vi "MotorBlock_PI.vi"(0 "P":dbl, 3 "STOP":bool, 5 "Value":dbl, 7 "Custom FPGA Reference Out":refnum<k20>, 9 "Speed\n (Lower than 900 counts/s)":dbl, 11 "error in (no error)":errorcluster, 12 "Enum":T2(ring), 13 "Motor":T1(ring), 14 "(Antihorario) Sentido (Horario)":bool) -> (4 "Waveform \nChart":dbl[][](graph), 10 "Custom FPGA Reference Out 2":refnum<k20>, 15 "error out":errorcluster)   [LabVIEW 2017]
uses:
  <vilib>/myRIO/Common/Instrument Driver Framework/myRIO v1.0/Encoder/typedefs/Encoder Signal Mode.ctl
  <vilib>/Platform/TimedLoop/XDataNode/timing_clust.ctl
  <vilib>/Platform/TimedLoop/XDataNode/nitl_modes.ctl
  <vilib>/Platform/TimedLoop/XDataNode/wakeup.ctl
  <vilib>/myRIO/Common/Instrument Driver Framework/myRIO v1.0/UART/vis/myRIO v1.0 Close UART.vi
  <vilib>/Utility/error.llb/Error Cluster From Error Code.vi
  <vilib>/myRIO/Common/Instrument Driver Framework/myRIO v1.0/Encoder/vis/myRIO v1.0 Read Encoder.vi
  <vilib>/myRIO/Common/Instrument Driver Framework/myRIO v1.0/DIO/vis/myRIO v1.0 Write DIO.vi
  <vilib>/myRIO/Common/Instrument Driver Framework/myRIO v1.0/PWM/vis/myRIO v1.0 Write PWM.vi
  <vilib>/myRIO/Common/Instrument Driver Framework/Utilities/vis/FPGA Ref Manager.vi
  <vilib>/myRIO/Common/Instrument Driver Framework/myRIO v1.0/myRIO v1.0 Reset FPGA.vi
  <vilib>/myRIO/Common/Instrument Driver Framework/myRIO v1.0/IRQ/vis/myRIO v1.0 IRQ Info FGV.vi
  <vilib>/myRIO/Common/Instrument Driver Framework/myRIO v1.0/IRQ/vis/myRIO v1.0 Timer IRQ Info FGV.vi
  <vilib>/myRIO/Common/Instrument Driver Framework/myRIO v1.0/IRQ/vis/myRIO v1.0 ISR Agent.vi
  <vilib>/Platform/TimedLoop/XDataNode/XDataNode.xnode
  <vilib>/myRIO/Instrument Drivers/Utilities/Utilities.lvlib
  <vilib>/myRIO/Instrument Drivers/Onboard IO/PWM/PWM.lvlib
  <vilib>/myRIO/Instrument Drivers/Onboard IO/DIO/DIO.lvlib
  <vilib>/myRIO/Instrument Drivers/Onboard IO/Encoder/Encoder.lvlib
  <vilib>/Platform/TimedLoop/XDataNode/XDNodeRunTimeDep.lvlib
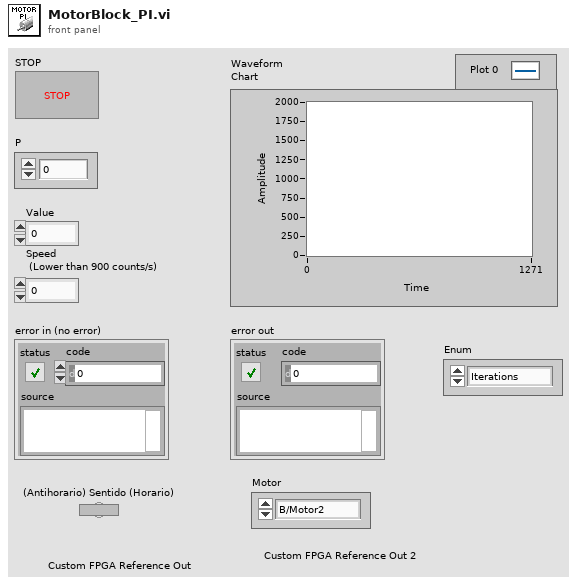
[diagram p1: front panel]
types:
  T1 = enum16{"B/Motor2", "B/Motor1", "A/Motor2", "A/Motor1"}
  T2 = enum16{"Iterations", "Rotations", "Counts", "Degrees", "Time"}
  T3 = typedef "Encoder Signal Mode.ctl" = enum16{"Quadrature phase signal", "Step and direction signal"}
  T4 = typedef "XDNodeRunTimeDep.lvlib/timing_clust.ctl" = cluster{"Expected End [f-1]":u64, "Actual End [f-1]":u64, "Finished Late? [f-1]":bool, "Expected End [i-1]":u64, "Actual End [i-1]":u64, "Finished Late? [i-1]":bool, "Expected Start [i]":u64, "Actual Start [i]":u64, "Expected Start [f]":u64, "Actual Start [f]":u64, "Source Name":string, "Structure Name":string, "Period":i64, "Deadline":i64, "Offset":i64, "Start":i64, "Priority":i32, "Timeout":i32, "Mode":T5, "Wakeup Reason":T6, "Error":errorcluster, "Source Type":string, "Secondary Source Type":string, "Global End Time":u64, "Global Start Time":u64, "Frame Duration":u64, "Iteration Duration":u64, "Assigned CPU":i32, "I/O Scan Engine Mode":u32}
  T5 = typedef "XDNodeRunTimeDep.lvlib/nitl_modes.ctl" = enum32{"No Change", "Process missed periods, maintain original phase", "Discard missed periods, maintain original phase", "Process missed periods, ignore original phase", "Discard missed periods, ignore original phase"}
  T6 = typedef "XDNodeRunTimeDep.lvlib/wakeup.ctl" = enum32{"Normal", "Aborted", "Asynchronous wakeup", "Timing source error", "Timed loop error", "Timeout"}
  T7 = typedef "Encoder.lvlib/Encoder Reference.ctl" = cluster{"myRIO Reference":T8, "Encoder Channels Enum":T12}
  T8 = typedef "myRIO Generic Hardware Reference.ctl" = cluster{"myRIO Model":T9, "myRIO Hardware Reference":T10}
  T9 = typedef "Hardware Version Enum.ctl" = enum16{"Unknown", "myRIO-1900", "myRIO-1950", "roboRIO", "NI ELVIS RIO CM"}
  T10 = typedef "myRIO v1.0 Reference.ctl" = cluster{"Generic FPGA Reference":T11, "Allow multiple opens":bool}
  T11 = typedef "Generic FPGA Reference.ctl" = refnum<k20>
  T12 = typedef "Encoder Channels Enum.ctl" = enum16{"Not Connected", "C/ENC0", "C/ENC1", "A/ENC", "B/ENC", "DIO/ENC0", "DIO/ENC1", "DIO/ENC2", "DIO/ENC3", "DIO/ENC4"}
  T13 = typedef "DIO.lvlib/DIO Reference.ctl" = cluster{"myRIO Reference":T8, "DIO Channels List":T14}
  T14 = typedef "DIO Channels List.ctl" = T15[]
  T15 = typedef "DIO Channels Enum.ctl" = enum16{"Not Connected", "C/DIO0", "C/DIO1", "C/DIO2", "C/DIO3", "C/DIO4", "C/DIO5", "C/DIO6", "C/DIO7", "A/DIO0", "A/DIO1", "A/DIO2", "A/DIO3", "A/DIO4", "A/DIO5", "A/DIO6", "A/DIO7", "A/DIO8", "A/DIO9", "A/DIO10", "A/DIO11", "A/DIO12", "A/DIO13", "A/DIO14", "A/DIO15", "B/DIO0", "B/DIO1", "B/DIO2", "B/DIO3", "B/DIO4", "B/DIO5", "B/DIO6", "B/DIO7", "B/DIO8", "B/DIO9", "B/DIO10", "B/DIO11", "B/DIO12", "B/DIO13", "B/DIO14", "B/DIO15", "LED0", "LED1", "LED2", "LED3", "Button0", "DIO/DIO0", "DIO/DIO1", "DIO/DIO2", "DIO/DIO3", "DIO/DIO4", "DIO/DIO5", "DIO/DIO6", "DIO/DIO7", "DIO/DIO8", "DIO/DIO9", "SPI/CS0", "SPI/CS1", "SPI/CS2", "SPI/CS3", "LED RADIO (Green)", "LED RADIO (Red)", "LED COMM (Green)", "LED COMM (Red)", "LED MODE (Green)", "LED MODE (Red)"}
  T16 = typedef "PWM.lvlib/PWM Reference.ctl" = cluster{"myRIO Reference":T8, "PWM Channels Enum":T17, "PWM Configuration":T18}
  T17 = typedef "PWM Channels Enum.ctl" = enum16{"Not Connected", "C/PWM0", "C/PWM1", "A/PWM0", "A/PWM1", "A/PWM2", "B/PWM0", "B/PWM1", "B/PWM2", "PWM/PWM0", "PWM/PWM1", "PWM/PWM2", "PWM/PWM3", "PWM/PWM4", "PWM/PWM5", "PWM/PWM6", "PWM/PWM7", "PWM/PWM8", "PWM/PWM9"}
  T18 = typedef "PWM.lvlib/PWM Configuration.ctl" = cluster{"Frequency":dbl, "Duty Cycle":dbl}
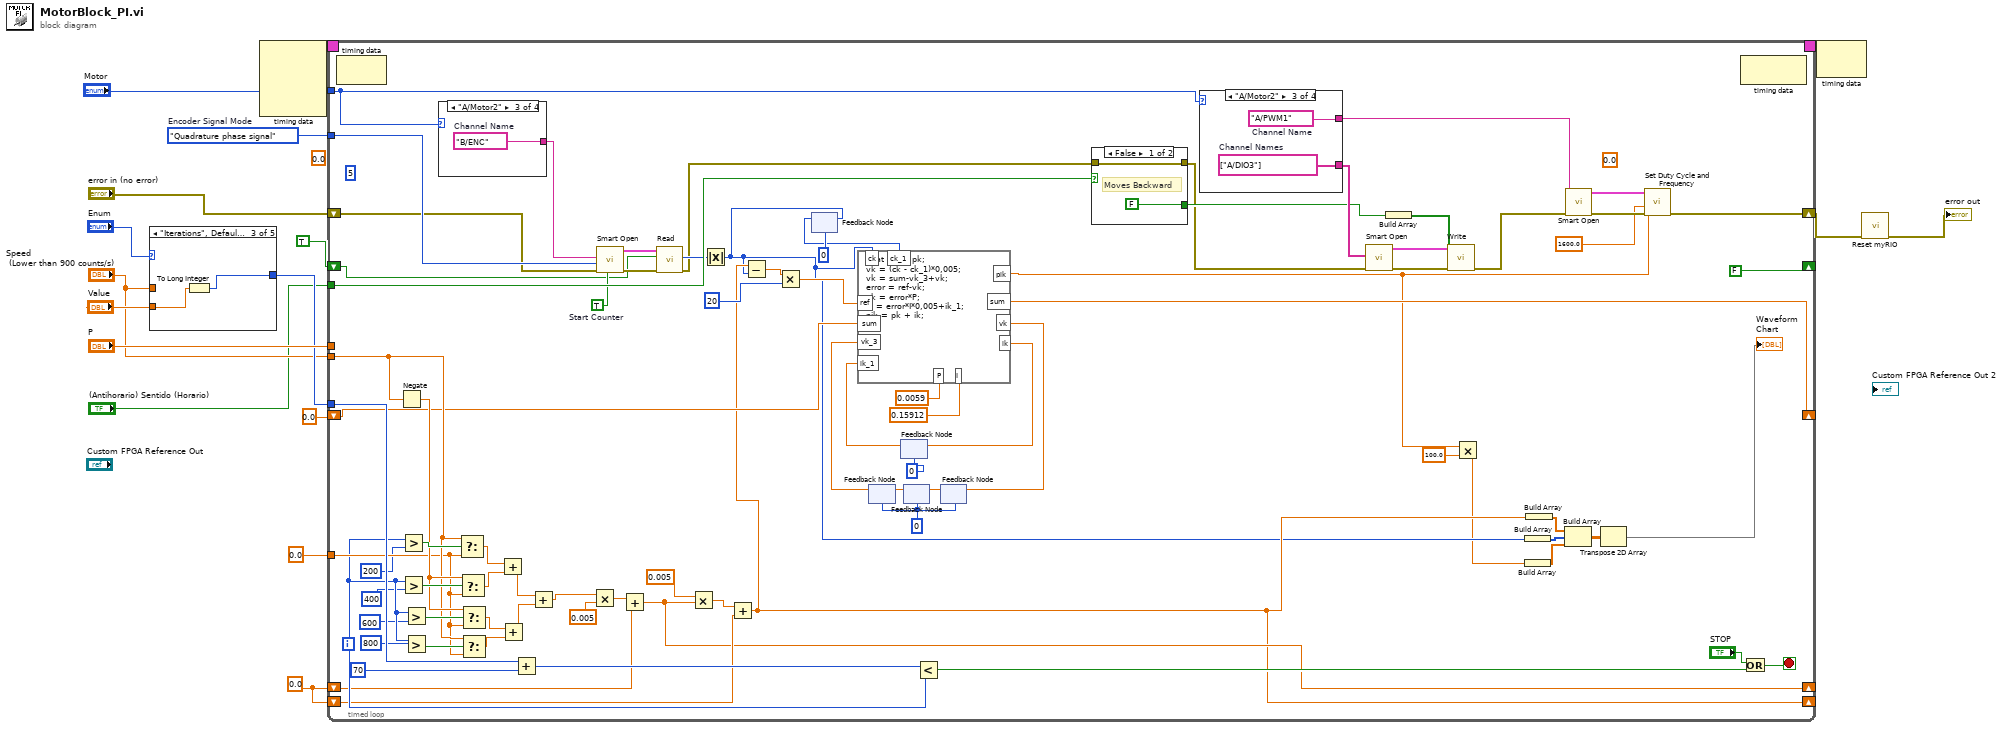
[diagram p0: block diagram]
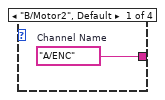
[diagram p2: hidden frame]
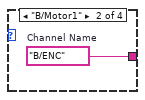
[diagram p3: hidden frame]
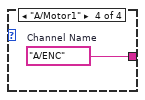
[diagram p4: hidden frame]
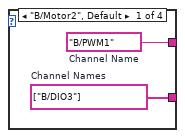
[diagram p5: hidden frame]
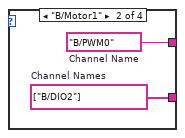
[diagram p6: hidden frame]
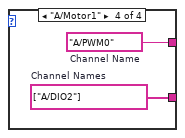
[diagram p7: hidden frame]
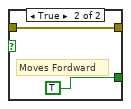
[diagram p8: hidden frame]
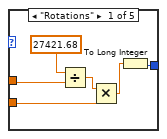
[diagram p9: hidden frame]
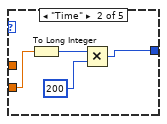
[diagram p10: hidden frame]
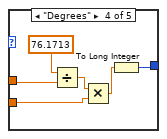
[diagram p11: hidden frame]
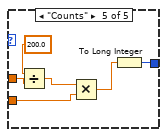
[diagram p12: hidden frame]
diagram:
  w1 = 0.0
  w5 = Encoder_Signal_Mode."Quadrature phase signal"  # Encoder Signal Mode
  (unwired) 0.0
  n1 = case shown="\"Iterations\", Default" "Enum" {
    tunnel: "Value" -> [w19 w24 w29 w30 w37]
    tunnel: "Speed\n (Lower than 900 counts/s)" -> [w20 _ _ w33 w40]
    tunnel: [w18 w26 w28 w35 w41] -> w11
    frame "Rotations" {
      n2 = Divide(x=27421.68 ("y"), y=w20) -> (x/y=w23:dbl)
      n3 = Multiply(x=w23, y=w19) -> (x*y=w21:dbl)
      n4 = To Long Integer(number=w21) -> (32bit integer=w18:i32)
    }
    frame "Time" {
      n5 = To Long Integer(number=w24) -> (32bit integer=w25:i32)
      n6 = Multiply(x=w25, y=200) -> (x*y=w26:i32)
    }
    frame "Iterations", Default {
      n7 = To Long Integer(number=w29) -> (32bit integer=w28:i32)
    }
    frame "Degrees" {
      n8 = Divide(x=76.1713 ("y"), y=w33) -> (x/y=w31:dbl)
      n9 = Multiply(x=w31, y=w30) -> (x*y=w34:dbl)
      n10 = To Long Integer(number=w34) -> (32bit integer=w35:i32)
    }
    frame "Counts" {
      n11 = Divide(x=200.0, y=w40) -> (x/y=w38:dbl)
      n12 = Multiply(x=w38, y=w37) -> (x*y=w36:dbl)
      n13 = To Long Integer(number=w36) -> (32bit integer=w41:i32)
    }
  }
  n14 = node-c288() -> (w4:T4)  [unwired: 4 in]
  n15 = timed-loop {
    shift-right: [w66] -> _
    shift-left: 0.0 -> [w65]
    shift-right: [FALSE] -> _
    shift-left: TRUE -> [w99]
    tunnel: "P" -> [_]
    tunnel: "Speed\n (Lower than 900 counts/s)" -> [w91]
    shift-right: [w112] -> w6
    shift-left: "error in (no error)" -> [w96]
    tunnel: w11 -> [w119]
    tunnel: "(Antihorario) Sentido (Horario)" -> [w123]
    tunnel: "Motor" -> [w101]
    tunnel: w5 -> [w97]
    timing: w4 -> [_]
    timing-out: [_] -> w3
    tunnel: 0.0 ("f") -> [w89]
    shift-right: [w52] -> _
    shift-left: w1 -> [w54]
    shift-right: [w47] -> _
    shift-left: w1 -> [w53]
    i -> [w77]
    stop <- w120 stop-if-true
    (unwired) 0.0 ("Duty Cycle")
    w72 = 0
    w104 = TRUE  # Start Counter
    (unwired) 5
    n16 = node-c288() -> ()  [unwired: 1 in, 1 out]
    n17 = Negate(x=w91) -> (-x=w93:dbl)
    n18 = Greater?(x=w77, y=200) -> (0:w95:bool)
    n19 = Greater?(x=w77, y=400) -> (0:w94:bool)
    n20 = Greater?(x=w77, y=600) -> (0:w92:bool)
    n21 = Greater?(x=w77, y=800) -> (0:w90:bool)
    n22 = case shown="\"A/Motor2\"" w101 {
      tunnel: [w127 w128 w129 w130] -> w100
      frame "B/Motor2", Default {
        w127 = tag "A/ENC"  # Channel Name
      }
      frame "B/Motor1" {
        w128 = tag "B/ENC"  # Channel Name
      }
      frame "A/Motor2" {
        w129 = tag "B/ENC"  # Channel Name
      }
      frame "A/Motor1" {
        w130 = tag "A/ENC"  # Channel Name
      }
    }
    n23 = Select(t=w91, s=w95, f=w89) -> (s? t:f=w88:dbl)
    n24 = Select(t=w93, s=w94, f=w89) -> (s? t:f=w87:dbl)
    n25 = Select(t=w93, s=w92, f=w89) -> (s? t:f=w86:dbl)
    n26 = Select(t=w91, s=w90, f=w89) -> (s? t:f=w85:dbl)
    n27 = Add(x=w88, y=w87) -> (x+y=w84:dbl)
    n28 = Add(x=w86, y=w85) -> (x+y=w83:dbl)
    n29 = Add(x=w119, y=70) -> (x+y=w117:i32)
    n30 = Add(x=w84, y=w83) -> (x+y=w82:dbl)
    n31 = Multiply(x=w82, y=0.005) -> (x*y=w80:dbl)
    n32 = call <vilib>:"Smart Open.vi"("Start Counter"=w104, "error in (no error)"=w96, "Encoder Signal Mode"=w97, "Channel Name"=w100) -> ("error out"=w102:errorcluster, "Encoder Ref Out"=w103:T7)  [unwired: 6 in]
    n33 = Add(x=w80, y=w54) -> (x+y=w52:dbl)
    n34 = call <vilib>:"Read.vi"("error in (no error)"=w102, "Reset Counter"=w99, "Encoder Ref In"=w103) -> ("error out"=w59:errorcluster, "Counter Value"=w98:i32)  [unwired: 4 in, 3 out]
    n35 = Multiply(x=0.005, y=w52) -> (x*y=w78:dbl)
    n36 = Absolute Value(x=w98) -> (abs(x)=w46:i32)
    n37 = Add(x=w78, y=w53) -> (x+y=w47:dbl)
    n38 = Subtract(x=w47, y=w46) -> (x-y=w61:dbl)
    n39 = Multiply(x=w61, y=20) -> (x*y=w60:dbl)
    n40 = feedback-in #1(w46) -> ()
    n41 = feedback #1(0) -> (w75:i32)
    n42 = feedback #2(w72) -> (w71:dbl)
    n43 = feedback #3(0) -> (w67:dbl)
    n44 = formula code="float error, pk;\nvk = (ck - ck_1)*0,005;\nvk = sum-vk_3+vk;\nerror = ref-vk;\npk = error*P;\nik = error*I*0,005+ik_1;\npik = pk + ik;"("ck"=w46, "ck_1"=w75, "sum"=w65, "vk_3"=w71, "ref"=w60, "I"=0.15912 ("input variable"), "P"=0.0059 ("input variable"), "ik_1"=w67) -> ("vk"=w70:dbl, "ik"=w69:dbl, "pik"=w44:dbl, "sum"=w66:dbl)
    n45 = feedback-in #3(w69) -> ()
    n46 = feedback #4(w72) -> (w73:dbl)
    n47 = feedback-in #2(w73) -> ()
    n48 = Less?(x=w117, y=w77) -> (x < y?=w121:bool)
    n49 = feedback-in #5(w70) -> ()
    n50 = feedback #5(w72) -> (w74:dbl)
    n51 = feedback-in #4(w74) -> ()
    n52 = case shown="False" w123 {
      tunnel: w59 -> [w139 w141]
      tunnel: [FALSE ("A/DIO3 (Pin 17)") TRUE ("A/DIO3 (Pin 17)")] -> w107
      tunnel: [w139 w141] -> w106
      frame False {
        # "Moves Backward"
      }
      frame True {
        # "Moves Fordward"
      }
    }
    n53 = case shown="\"A/Motor2\"" w101 {
      tunnel: [w131 w134 w135 w138] -> w114
      tunnel: [w132 w133 w136 w137] -> w108
      frame "B/Motor2", Default {
        w132 = tag[] ["B/DIO3"]  # Channel Names
        w131 = tag "B/PWM1"  # Channel Name
      }
      frame "B/Motor1" {
        w133 = tag[] ["B/DIO2"]  # Channel Names
        w134 = tag "B/PWM0"  # Channel Name
      }
      frame "A/Motor2" {
        w136 = tag[] ["A/DIO3"]  # Channel Names
        w135 = tag "A/PWM1"  # Channel Name
      }
      frame "A/Motor1" {
        w137 = tag[] ["A/DIO2"]  # Channel Names
        w138 = tag "A/PWM0"  # Channel Name
      }
    }
    n54 = call <vilib>:"Smart Open.vi"("error in (no error)"=w106, "Channel Names"=w108) -> ("error out"=w111:errorcluster, "DIO Ref Out"=w110:T13)  [unwired: 8 in]
    n55 = Build Array(w107) -> (w109:bool[])
    n56 = call <vilib>:"Write.vi"("error in (no error)"=w111, "Values"=w109, "DIO Ref In"=w110) -> ("error out"=w105:errorcluster)  [unwired: 6 in, 1 out]
    n57 = Multiply(x=w44, y=100.0) -> (x*y=w42:dbl)
    n58 = Build Array(w46) -> (w49:i32[])
    n59 = Build Array(w42) -> (w48:dbl[])
    n60 = Build Array(w47) -> (w50:dbl[])
    n61 = Build Array(w50, w49, w48) -> (w51:dbl[][])
    n62 = call <vilib>:"Smart Open.vi"("error in (no error)"=w105, "Channel Name"=w114) -> ("error out"=w115:errorcluster, "PWM Ref Out"=w116:T16)  [unwired: 8 in]
    n63 = Transpose 2D Array(2D array=w51) -> (transposed array=→"Waveform \nChart":dbl[][])
    n64 = call <vilib>:"Set Duty Cycle and Frequency.vi"("error in (no error)"=w115, "Frequency [Hz]"=1600.0 ("Duty Cycle"), "Duty Cycle"=w44, "PWM Ref In"=w116) -> ("error out"=w112:errorcluster)  [unwired: 5 in, 1 out]
    n65 = node-c288() -> ()  [unwired: 1 in, 1 out]
    n66 = Or(x="STOP", y=w121) -> (x .or. y?=w120:bool)
  }
  n67 = node-c288(w3) -> ()  [unwired: 1 out]
  n68 = call <vilib>:"Reset myRIO.vi"("error in (no error)"=w6) -> ("error out"=→"error out":errorcluster)  [unwired: 10 in]
